vi "Detect QR Codes (ARGB).vi"(8 "error in (no error)":errorcluster, 10 "ARGB Image":T4, 11 "QR Code Detector in":refnum<class "QR Code Detector.lvclass">) -> (0 "error out":errorcluster, 2 "Detections":T1[](array[typedef]), 3 "QR Code Detector (Duplicate)":refnum<class "QR Code Detector.lvclass">)   [LabVIEW 2020, in "feature_detection.lvlib" / "QR Code Detector.lvclass"]
uses:
  QR Code Detector.lvclass
  image/ARGB Image.ctl
  Detection.ctl
  Detection Region.ctl
  common/Image Point (Float).ctl
  QR Code Detector.lvclass/QR Code Detector.ctl
  947807d6-cf22-42cc-b024-3c0d53b5d2ed.vi
  common/Module Path.vi
  <vilib>/Utility/error.llb/Error Cluster From Error Code.vi
  common/common.lvlib
  image/image.lvlib
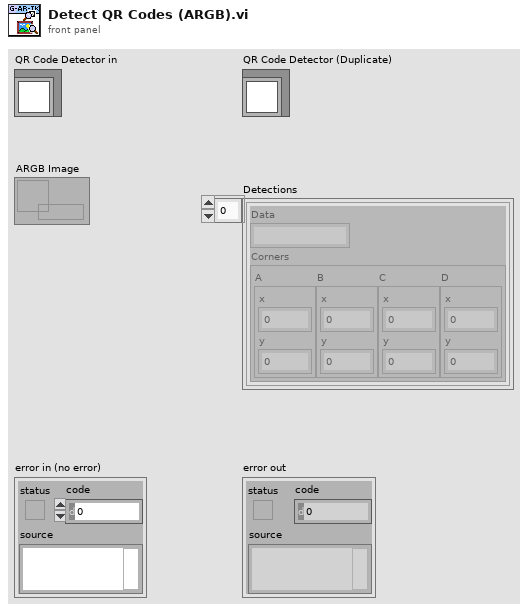
[diagram p1: front panel]
types:
  T1 = typedef "feature_detection.lvlib/QR Code Detector.lvclass/Detection.ctl" = cluster{"Data":string, "Corners":T2}
  T2 = typedef "feature_detection.lvlib/QR Code Detector.lvclass/Detection Region.ctl" = cluster{"A":T3, "B":T3, "C":T3, "D":T3}
  T3 = typedef "common.lvlib/Image Point (Float).ctl" = cluster{"x":dbl, "y":dbl}
  T4 = typedef "image.lvlib/ARGB Image.ctl" = refnum<data-value>
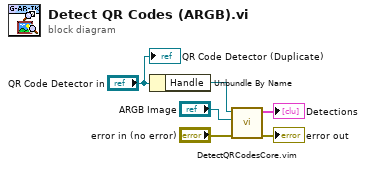
[diagram p0: block diagram]
diagram:
  n1 = Unbundle By Name("QR Code Detector in") -> ("Handle"=w1:refnum<data-value>)
  n2 = call "DetectQRCodesCore.vim"("error in (no error)"="error in (no error)", "Greyscale Image"="ARGB Image", "Handle"=w1) -> ("error out"=→"error out":errorcluster, "Detections"=→"Detections":T1[])  [unwired: 7 in]
  "QR Code Detector (Duplicate)" <- "QR Code Detector in"
